vi "FIR_5interpolate_10cycles.vi"(7 "reset":bool, 8 "valid in":bool, 10 "Q in":fxp<+/-,16,14>, 11 "I in":fxp<+/-,16,14>) -> (0 "valid out":bool, 2 "Q out":fxp<+/-,16,14>, 3 "I out":fxp<+/-,16,14>, 4 "ready for input":bool)   [LabVIEW 2013]
uses:
  <vilib>/rvi/FXPMathLib/FxpConvert/subVIs/nifxpmath_Convert_SimConfig.ctl
  <vilib>/fxp/LVFixedPointQuantizationPolicyTypeDef.ctl
  <vilib>/fxp/LVFixedPointOverflowPolicyTypeDef.ctl
  <vilib>/rvi/IPIntegrationNode/IPINode_Utilities/niFpgaIPINodeSimCore.vi
  <vilib>/rvi/FXPMathLib/FxpConvert/simVIs/DllFxpConvertTemp_sub.vi
  <vilib>/rvi/XilinxIP/XIPIN_XNode/niFpgaXIPIN.xnode
  FIR_5interpolate_10cycles/FIR Compiler/FIR_Compiler_5FB9F0BADE11496F8820C1DDE59652D9.dll
  <vilib>/rvi/IPIntegrationNode/IPINode_Xnode/niFpgaIPINode.xnode
  <vilib>/rvi/FXPMathLib/FxpInterpret/XNode/nifxpmath_Interpret.xnode
  <vilib>/rvi/FXPMathLib/FxpConvert/XNode/nifxpmath_Convert.xnode
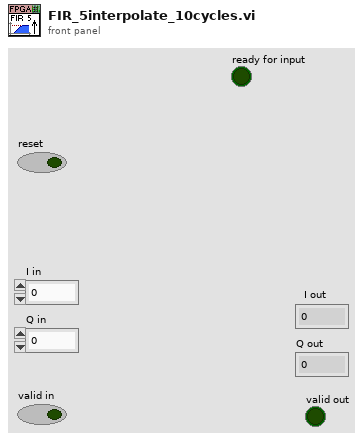
[diagram p1: front panel]
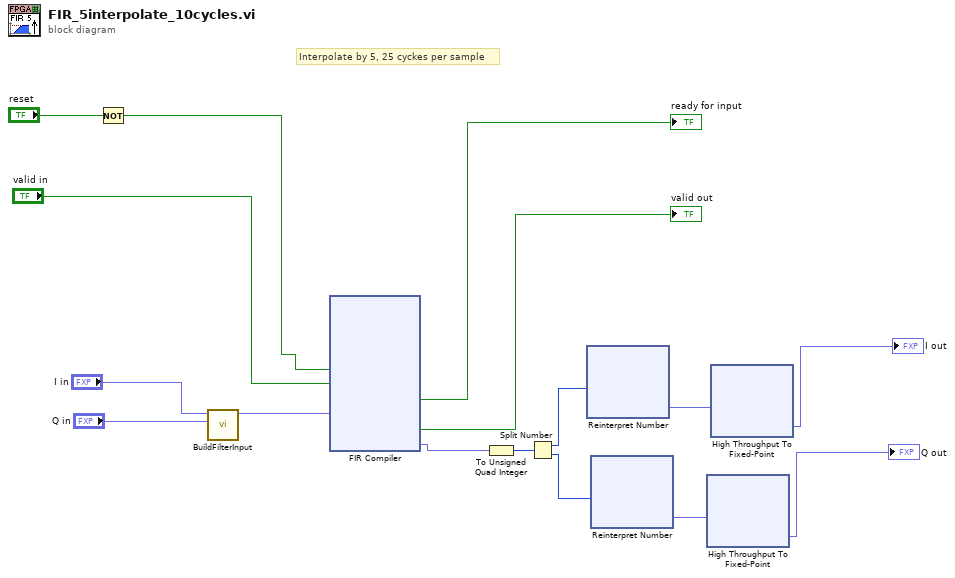
[diagram p0: block diagram]
diagram:
  # "Interpolate by 5, 25 cyckes per sample"
  n1 = Not(x="reset") -> (.not. x?=w6:bool)
  n2 = call "BuildFilterInput.vi"("Q in"="Q in", "I in"="I in") -> ("Filter input"=w4:fxp<+,32,32>)  [unwired: 9 in]
  n3 = xnode ("FIR Compiler")("aresetn"=w6, "s_axis_data_tvalid"="valid in", "s_axis_data_tdata"=w4) -> ("s_axis_data_tready"=→"ready for input":bool, "m_axis_data_tvalid"=→"valid out":bool, "m_axis_data_tdata"=w1:fxp<+,64,64>)  [unwired: 1 in]
  n4 = To Unsigned Quad Integer(1:w1) -> (0:w12:u64)
  n5 = Split Number(x=w12) -> (hi(x)=w13:u32, lo(x)=w9:u32)
  n6 = xnode "Reinterpret Number"("x"=w13) -> ("y"=w10:fxp<+/-,32,16>)
  n7 = xnode "Reinterpret Number"("x"=w9) -> ("y"=w11:fxp<+/-,32,16>)
  n8 = xnode "High Throughput To Fixed-Point"("x"=w11) -> ("y"=→"Q out":fxp<+/-,16,14>)
  n9 = xnode "High Throughput To Fixed-Point"("x"=w10) -> ("y"=→"I out":fxp<+/-,16,14>)
